vi "Handshake Startup.vi"(7 "Startup Notifier":refnum<notifier>, 8 "error in (no error)":errorcluster, 11 "BetterSearch in":refnum<class "BetterSearch.lvclass">) -> (0 "error out":errorcluster, 3 "BetterSearch out":refnum<class "BetterSearch.lvclass">)   [LabVIEW 2016, in "Better Search.lvlib" / "BetterSearch.lvclass"]
uses:
  BetterSearch.lvclass
  Data Types/Search Context.ctl
  Better Search.lvlib
  Data Types/Context Comms.ctl
  Data Types/Start Search Type.ctl
  Data Types/Type Reflection Item.ctl
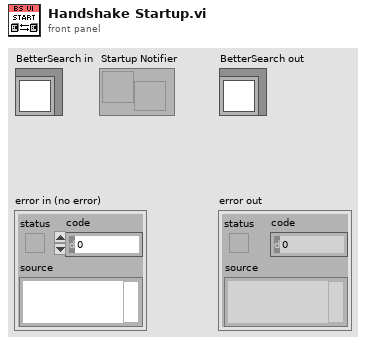
[diagram p1: front panel]
types:
  T1 = typedef "Better Search.lvlib/Context Comms.ctl" = cluster{"Context":refnum<user-event>, "Handshake":refnum<notifier>}
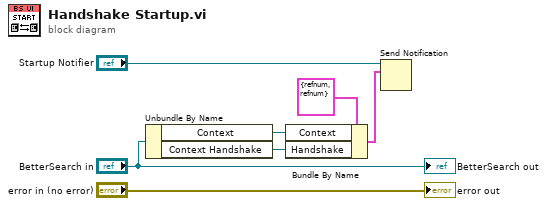
[diagram p0: block diagram]
diagram:
  n1 = Unbundle By Name("BetterSearch in") -> ("Context"=w4:refnum<user-event>, "Context Handshake"=w3:refnum<notifier>)
  n2 = Bundle By Name(cluster=T1 {"Context"=refnum, "Handshake"=refnum} ("Context Comms"), "Context"=w4, "Handshake"=w3) -> (w1:T1)
  n3 = Send Notification(notification=w1, notifier="Startup Notifier") -> ()  [unwired: 1 in, 2 out]
  "error out" <- "error in (no error)"
  "BetterSearch out" <- "BetterSearch in"
